vi "IO_Test_18V7.vi"() -> ()   [LabVIEW 2024]
uses:
  <vilib>/Instr/_visa.llb/VISA Configure Serial Port (Instr).vi
panel:
  in  "Send Speed":bool
  in  "Write Buffer":string
  in  "Fill!Drain":bool
  in  "Speed":i8(slide) scale=0.0..100.0
  out "Status":bool[](array[boolean])
  out "x = y?":bool
  out "read buffer ASC":string
  in  "Send":bool
  in  "stop":bool
  # "Fill"
  # "• Bit 0: Safe Start Violation\n• Bit 1: Required Channel Invalid\n• Bit 2: Serial Error\n• Bit 3: Command Timeout\n• Bit 4: Limit/Kill Switch\n• Bit 5: Low VIN\n• Bit 6: High VIN\n• Bit 7: Over Temperature\n• Bit 8: Motor Driver Error\n• Bit 9: ERR Line High"
  # "Drain"
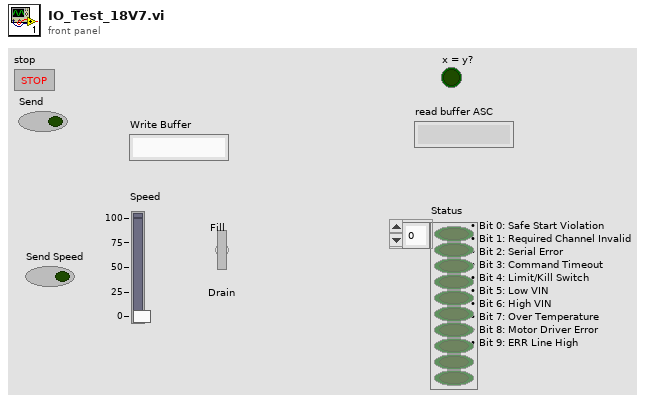
[diagram p1: front panel]
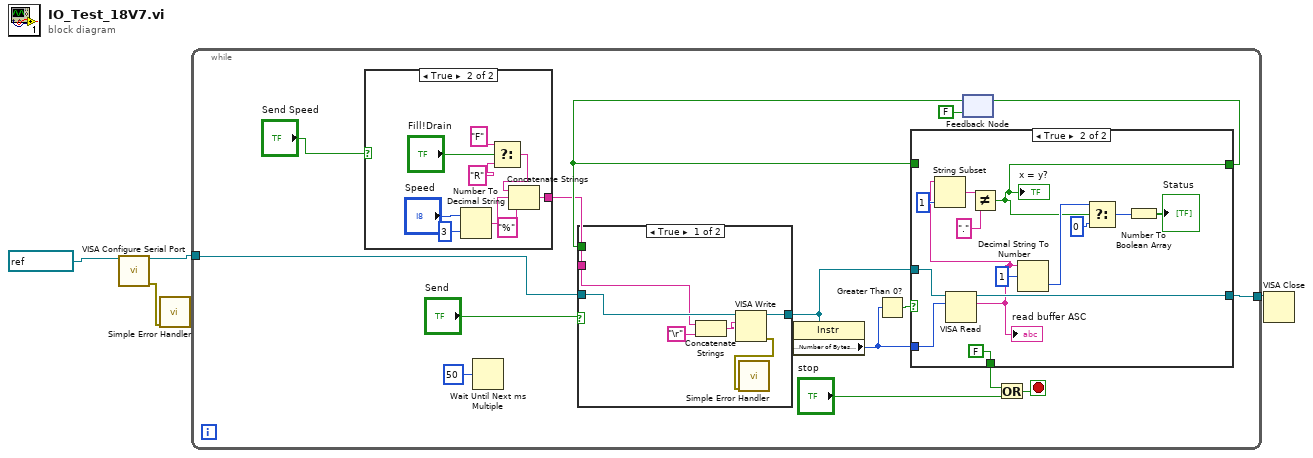
[diagram p0: block diagram]
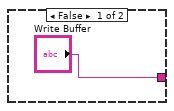
[diagram p2: hidden frame]
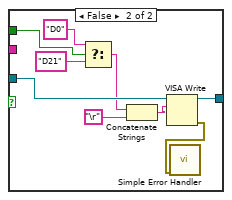
[diagram p3: hidden frame]
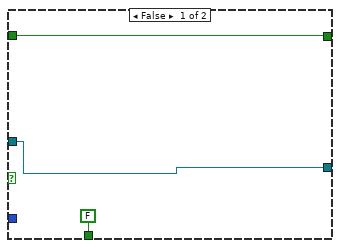
[diagram p4: hidden frame]
diagram:
  n1 = call-poly "VISA Configure Serial Port"("VISA resource name"=refnum<visa-resource-name> "COM4") -> ("VISA resource name out"=w2:refnum<visa-resource-name>, "error out"=w1:errorcluster)  [unwired: 13 in]
  n2 = call <vilib>:"Simple Error Handler.vi"("error in (no error)"=w1) -> ()  [unwired: 4 in, 5 out]
  n3 = while {
    tunnel: [w17] -> w4
    tunnel: w2 -> [w12]
    stop <- w16 stop-if-true
    n4 = case shown="True" "Send Speed" {
      tunnel: ["Write Buffer" w21] -> w6
      frame False {
      }
      frame True {
        n5 = Number To Decimal String(number="Speed", width (-)=i16 3) -> (decimal integer string=w23:string)
        n6 = Select(t="F", s="Fill!Drain", f="R") -> (s? t:f=w24:string)
        n7 = Concatenate Strings(w24, w23, "%" ("string")) -> (w21:string)
      }
    }
    n8 = Wait Until Next ms Multiple(millisecond multiple=u32 50) -> ()  [unwired: 1 out]
    n9 = feedback #1(FALSE) -> (w7:bool)
    n10 = case shown="True" "Send" {
      tunnel: w12 -> [w35 w44]
      tunnel: [w34 w43] -> w11
      tunnel: w7 -> [_ w37]
      tunnel: w6 -> [w30 _]
      frame True {
        n11 = Concatenate Strings(w30, "\r") -> (w33:string)
        n12 = VISA Write(VISA resource name=w35, write buffer=w33) -> (VISA resource name out=w34:refnum<visa-resource-name>, error out=w31:errorcluster)  [unwired: 1 in, 1 out]
        n13 = call <vilib>:"Simple Error Handler.vi"("error in (no error)"=w31) -> ()  [unwired: 4 in, 5 out]
      }
      frame False {
        n14 = Select(t="D0" ("write buffer 2"), s=w37, f="D21" ("write buffer 2")) -> (s? t:f=w36:string)
        n15 = Concatenate Strings(w36, "\r") -> (w42:string)
        n16 = VISA Write(VISA resource name=w44, write buffer=w42) -> (VISA resource name out=w43:refnum<visa-resource-name>, error out=w40:errorcluster)  [unwired: 1 in, 1 out]
        n17 = call <vilib>:"Simple Error Handler.vi"("error in (no error)"=w40) -> ()  [unwired: 4 in, 5 out]
      }
    }
    n18 = property class="Instr"(reference=w11) -> ("Serial Settings:Number of Bytes at Serial Port"=w18:u32)  [unwired: 1 in, 2 out]
    n19 = Greater Than 0?(x=w18) -> (x > 0?=w19:bool)
    n20 = case shown="True" w19 {
      tunnel: w11 -> [w46 w61]
      tunnel: w18 -> [_ w60]
      tunnel: [w46 w59] -> w17
      tunnel: [FALSE FALSE] -> w14
      tunnel: [w45 w49] -> w9
      tunnel: w7 -> [w45 _]
      frame False {
      }
      frame True {
        n21 = VISA Read(VISA resource name=w61, byte count=w60) -> (VISA resource name out=w59:refnum<visa-resource-name>, read buffer=w55:string)  [unwired: 1 in, 2 out]
        "read buffer ASC" <- w55
        n22 = String Subset(string=w55, length (rest)=1 ("length (rest)")) -> (substring=w54:string)  [unwired: 1 in]
        n23 = Not Equal?(x=w54, y=".") -> (x != y?=w49:bool)
        "x = y?" <- w49
        n24 = Decimal String To Number(string=w55, offset=1) -> (number=w50:i32)  [unwired: 1 in, 1 out]
        n25 = Select(t=w50, s=w49, f=0) -> (s? t:f=w51:i32)
        n26 = Number To Boolean Array(number=w51) -> (Boolean array=→"Status":bool[])
      }
    }
    n27 = feedback-in #1(w9) -> ()
    n28 = Or(x=w14, y="stop") -> (x .or. y?=w16:bool)
  }
  n29 = VISA Close(VISA resource name=w4) -> ()  [unwired: 1 in, 1 out]
